vi "Process.vi"(8 "error in":errorcluster, 11 "Inst UI.Krohn-Hite-7008":refnum<class "Inst UI.Krohn-Hite-7008.lvclass">) -> (0 "error out":errorcluster, 3 "Inst UI.Krohn-Hite-7008 out":refnum<class "Inst UI.Krohn-Hite-7008.lvclass">)   [LabVIEW 2019, in "Inst.KH7008.lvlib" / "Inst UI.Krohn-Hite-7008.lvclass"]
doc: "---------------------------------------------------------------\nJKI State Machine Objects™\nhttp://jki.net/state-machine-objects/\nCopyright (C) 2005-2015, JKI <info@jki.net>\nALL RIGHTS RESERVEDJKI State Machine Objects (SMO) 1.0.0.5\nJKI - JKI\nCopyright (c) 2016, JKI"
uses:
  Inst UI.Krohn-Hite-7008.lvclass
  C:/Program Files/National Instruments/LabVIEW 2019/vi.lib/JKI/JKI SMO/SMO/SMO.lvclass
  C:/Program Files/National Instruments/LabVIEW 2019/user.lib/LevyLab/Instrument Framework/Instrument UI/Instrument UI.lvclass
  C:/Program Files/National Instruments/LabVIEW 2019/vi.lib/JKI/JKI SMO/SMO.UI/SMO.UI.lvclass
  KH7008/typedefs/allChannelProperties--Array.ctl
  KH7008/typedefs/channelProperties--Cluster.ctl
  KH7008/typedefs/channel--numeric.ctl
  KH7008/typedefs/gain--enum.ctl
  KH7008/typedefs/Input--Enum.ctl
  KH7008/typedefs/shunt--enum.ctl
  KH7008/typedefs/couple--Enum.ctl
  KH7008/typedefs/Filter--Enum.ctl
  Inst.Krohn-Hite-7008/Typedefs/setAllChannelsRequest--Cluster.ctl
  Inst.Krohn-Hite-7008/Inst.Krohn-Hite-7008.lvclass
  C:/Program Files/National Instruments/LabVIEW 2019/user.lib/LevyLab/Instrument Framework/Instrument/Instrument.lvclass
  <userlib>/LevyLab/Configuration/Configuration.lvclass
  <userlib>/LevyLab/RemoteControl/RemoteControl/Typedefs/Message--Cluster.ctl
  Inst.Krohn-Hite-7008/Typedefs/Inst.KH7008.device--Cluster.ctl
  <userlib>/LevyLab/Instrument Framework/Instrument UI/Instrument UI.lvclass/Instrument UI.ctl
  Inst UI.KH7008.UI--Cluster.ctl
  Inst.Krohn-Hite-7008/Typedefs/Inst.KH7008.getAll--Cluster.ctl
  Inst.Krohn-Hite-7008/Typedefs/getAllChannelsResponse--Cluster.ctl
  Inst.Krohn-Hite-7008/Inst.Krohn-Hite-7008.lvclass/Inst.Krohn-Hite-7008.ctl
  <vilib>/JKI/JKI SMO/SMO/SMO.lvclass/SMO.ctl
  <userlib>/LevyLab/Configuration/Configuration.lvclass/Configuration.ctl
  <userlib>/LevyLab/Instrument Framework/Instrument/Typedefs/Client Type--Enum.ctl
  <userlib>/LevyLab/Instrument Framework/Instrument/Instrument.lvclass/Instrument.ctl
  05e2a320-c8bb-41b2-9e77-26c6b753b84f.vi
  05e2a320-c8bb-41b2-9e77-26c6b753b84f.vi/d1df4cf9-d74a-44fa-a3ad-a094c8633207.vi
  05e2a320-c8bb-41b2-9e77-26c6b753b84f.vi/ff02851b-1958-46bb-bf4c-5be60d5017db.vi
  <vilib>/JKI/JKI SMO/SMO/Private/ReftoDVR--SMO.vi
  <vilib>/Utility/Data Type/Get Type Information.vi
  <vilib>/JDP Science/JSONtext/JSON text to Variant.vi
  <userlib>/LevyLab/Instrument Framework/Instrument/API/Instrument.sendMessageToProcess (variant).vi
  <vilib>/JDP Science/JSONtext/LVClass Serializer/JSONtext LVClass Serializer.lvclass
  <userlib>/LevyLab/Instrument Framework/Instrument/Instrument.lvclass
  <userlib>/LevyLab/Instrument Framework/Instrument UI/Instrument UI.lvclass
  <userlib>/LevyLab/RemoteControl/RemoteControl/RemoteControl.lvclass
  KH7008/KH7008.lvlib
  <vilib>/JKI/JKI SMO/SMO.UI/SMO.UI.lvclass
  <vilib>/JKI/JKI SMO/SMO/SMO.lvclass
  C:/Program Files/National Instruments/LabVIEW 2019/user.lib/LevyLab/Instrument Framework/Instrument Types/Amplifier/Instrument.Amplifier.lvclass
panel:
  out "String":string
  out "Slide":i32(slide) scale=0.0..60000.0
  in  "Cancel":bool
  in  "allChannelProperties":T1 {"channel" min=1 max=8 step=1}
  out "device":string
  out "Numeric":u32
  in  "Update":bool
  in  "STOP":bool
  # "SMO UI Template"
  # "For instructions on how to use the JKI State Machine Objects, examples and video tutorials, visit:\nhttp://jki.net/state-machine-objects/\n\nJKI State Machine Objects™\nhttp://jki.net/state-machine-objects/\nCopyright (C) 2005-2015, JKI <info@jki.net>\nALL RIGHTS RESERVED"
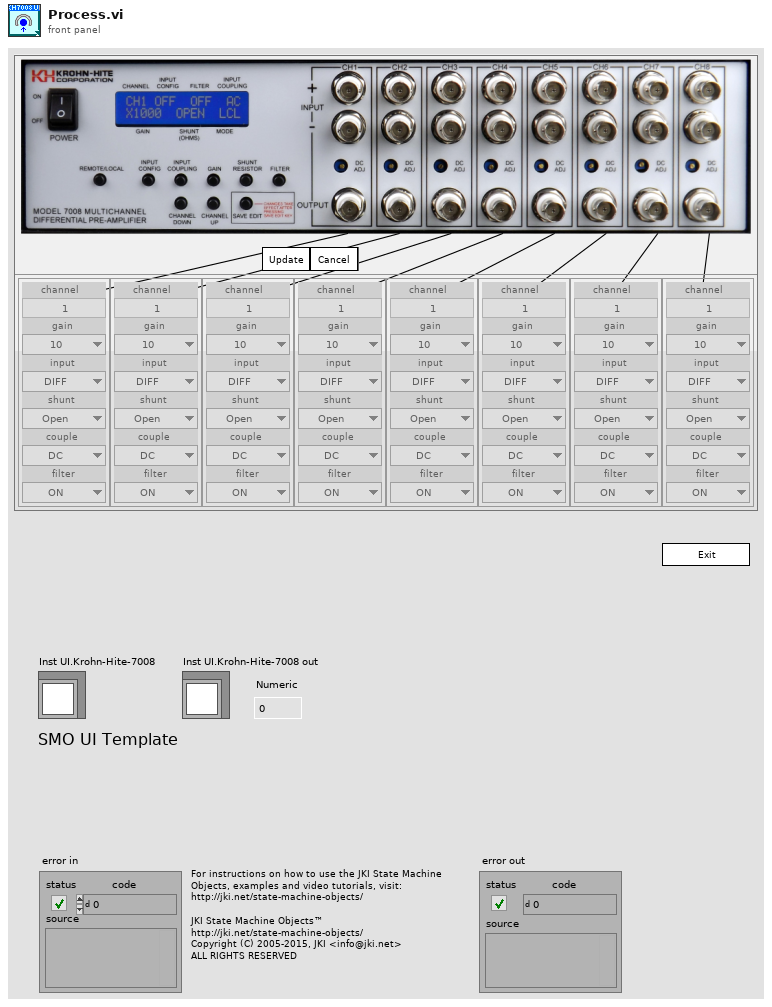
[diagram p1: front panel]
types:
  T1 = typedef "KH7008.lvlib/allChannelProperties--Array.ctl" = T2[]
  T2 = typedef "KH7008.lvlib/channelProperties--Cluster.ctl" = cluster{"channel":T3, "gain":T4, "input":T5, "shunt":T6, "couple":T7, "filter":T8}
  T3 = typedef "KH7008.lvlib/channel--numeric.ctl" = u16
  T4 = typedef "KH7008.lvlib/gain--enum.ctl" = enum16{"1", "10", "100", "1000"}
  T5 = typedef "KH7008.lvlib/input--enum.ctl" = enum16{"OFF", "SE+", "SE-", "DIFF"}
  T6 = typedef "KH7008.lvlib/shunt--enum.ctl" = enum16{"Open", "50", "500", "5k", "50k", "10M"}
  T7 = typedef "KH7008.lvlib/couple--enum.ctl" = enum16{"AC", "DC"}
  T8 = typedef "KH7008.lvlib/filter--enum.ctl" = enum16{"OFF", "ON"}
  T9 = typedef "Inst.KH7008.lvlib/Inst.Krohn-Hite-7008.lvclass/setAllChannelsRequest--Cluster.ctl" = cluster{"allChannelProperties":T1}
  T10 = enum32{"invalid app kind", "Development System", "Run Time System", "Student Edition", "Embedded LabVIEW", "Evaluation", "Custom"}
  T11 = typedef "Inst.KH7008.lvlib/Inst.Krohn-Hite-7008.lvclass/getAllChannelsResponse--Cluster.ctl" = cluster{"allChannelProperties":T1}
  T12 = enum32{"Invalid", "Standard", "Closed", "Hidden", "Minimized", "Maximized"}
  T13 = typedef "Instrument.lvlib/Instrument.lvclass/Client Type--Enum.ctl" = enum16{"Remote", "Local"}
  T14 = typedef "RemoteControl.lvlib/RemoteControl.lvclass/Message--Cluster.ctl" = cluster{"Command":string, "Data":variant, "ID":string}
  T15 = typedef "Inst.KH7008.lvlib/Inst.Krohn-Hite-7008.lvclass/Inst.KH7008.device--Cluster.ctl" = cluster{"model":string, "device_id":string, "index":i32}
  T16 = cluster{"Core":cluster{"Current VI Reference":refnum<vi>, "Close Panel on Exit?":bool, "Last Error":cluster{"error":errorcluster, "previous state":string, "remaining states":string}, "Shutdown?":bool}, "Instrument UI":refnum<class "Inst UI.Krohn-Hite-7008.lvclass">, "Instrument":refnum<class "Inst.Krohn-Hite-7008.lvclass">, "Configuration":refnum<class "Configuration.lvclass">, "Message":T14, "allChannelProperties":T1, "Device":T15, "Edit State":bool, "Timer Reset":bool}
  T17 = typedef "RemoteControl.lvclass/Message--Cluster.ctl" = cluster{"Command":string, "Data":variant, "ID":string}
  T18 = typedef "Inst.KH7008.lvlib/Inst.Krohn-Hite-7008.lvclass/Inst.KH7008.getAll--Cluster.ctl" = cluster{"allChannelProperties":T1}
  T19 = typedef "Inst.KH7008.lvlib/Inst UI.Krohn-Hite-7008.lvclass/Inst UI.KH7008.UI--Cluster.ctl" = cluster{"setAllChannelsRequest":T9}
  T20 = cluster{"Current VI Reference":refnum<vi>, "Close Panel on Exit?":bool, "Last Error":cluster{"error":errorcluster, "previous state":string, "remaining states":string}, "Shutdown?":bool}
  T21 = typedef "SMO.lvclass/Protected Events.ctl" = cluster{"StopProcesses":refnum<user-event>, "AbortProcesses":refnum<user-event>, "Config Changed":refnum<user-event>, "Dependency":refnum<user-event>}
  T22 = typedef "Instrument.lvlib/Instrument.lvclass/PublicEvents--Cluster.ctl" = cluster{"MessageFromProcess":refnum<user-event>}
  T23 = typedef "Inst.KH7008.lvlib/Inst.Krohn-Hite-7008.lvclass/PublicEvents--Cluster.ctl" = cluster{"MessageFromProcess":refnum<user-event>}
  T24 = typedef "Instrument.lvlib/Instrument.lvclass/Instrument.IDN--cluster.ctl" = cluster{"vendor":string, "model":string, "serial":string, "firmware":string}
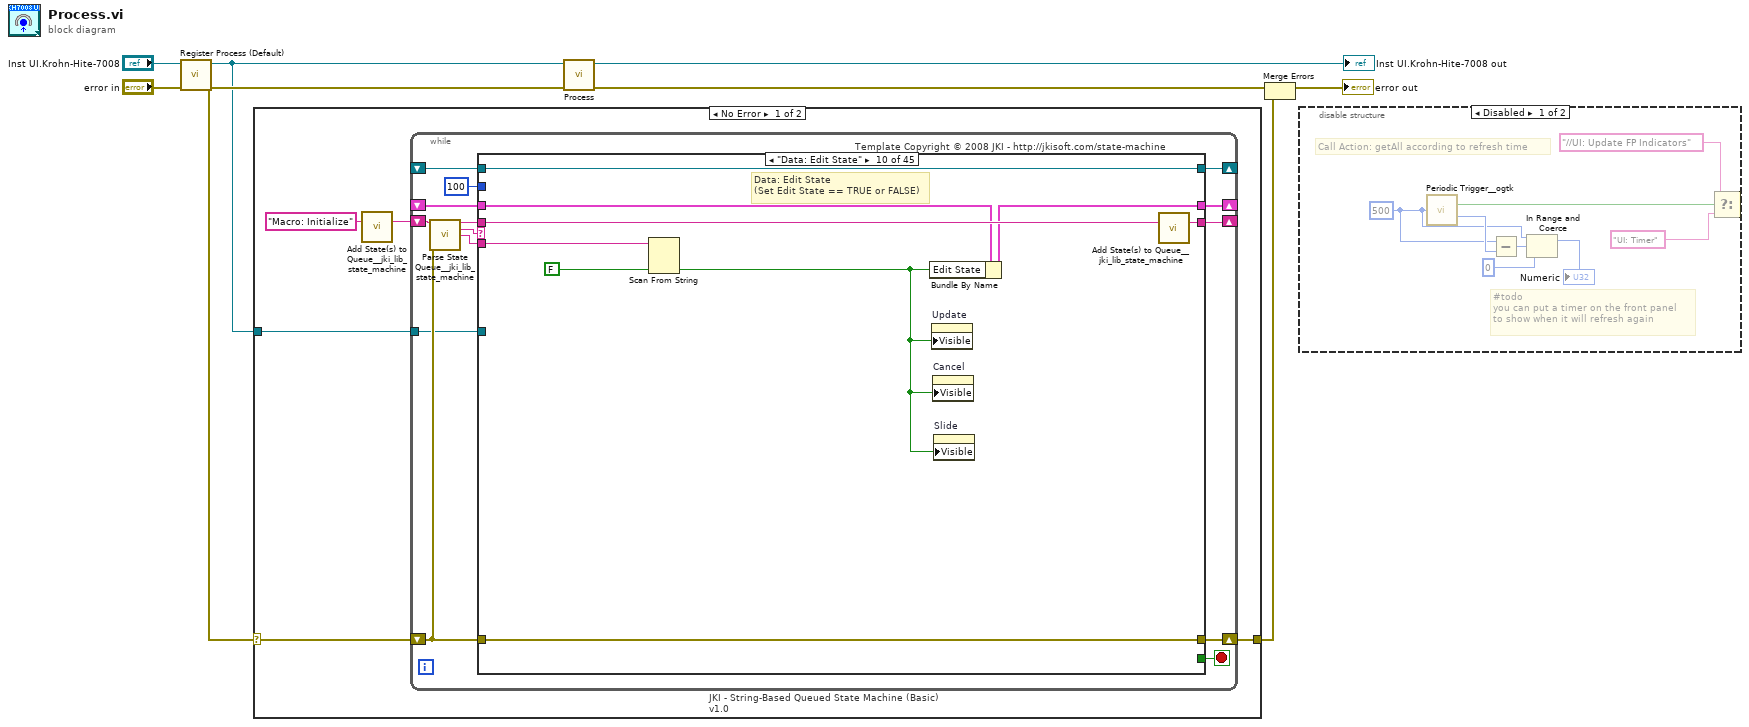
[diagram p0: block diagram]
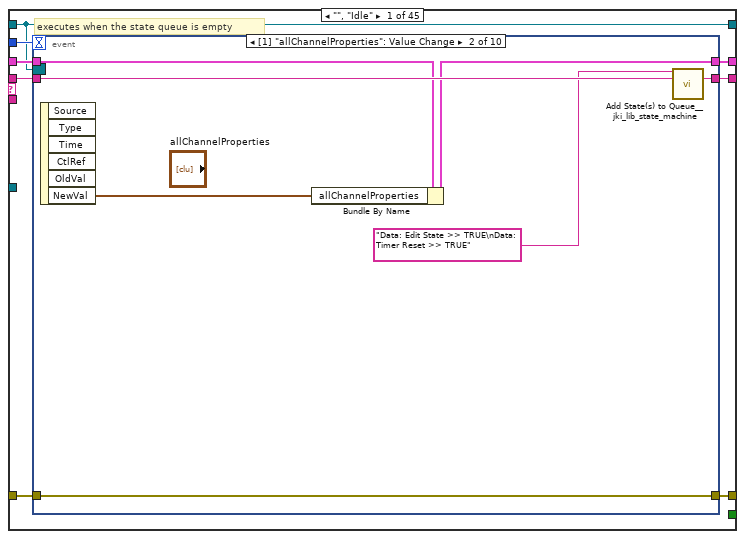
[diagram p3: hidden frame]
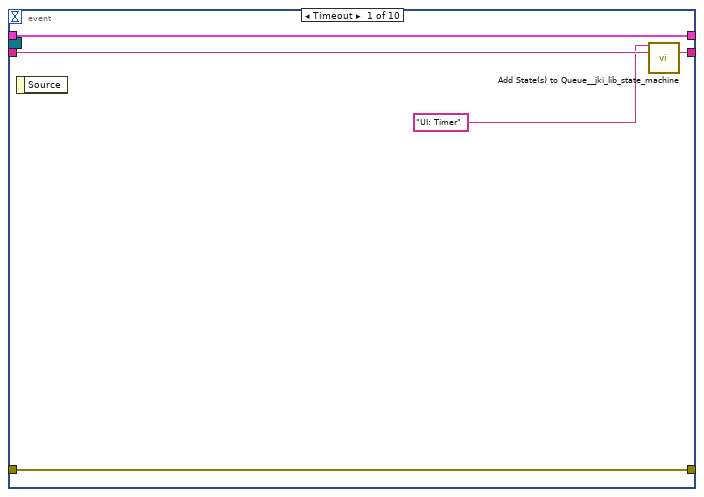
[diagram p4: hidden frame]
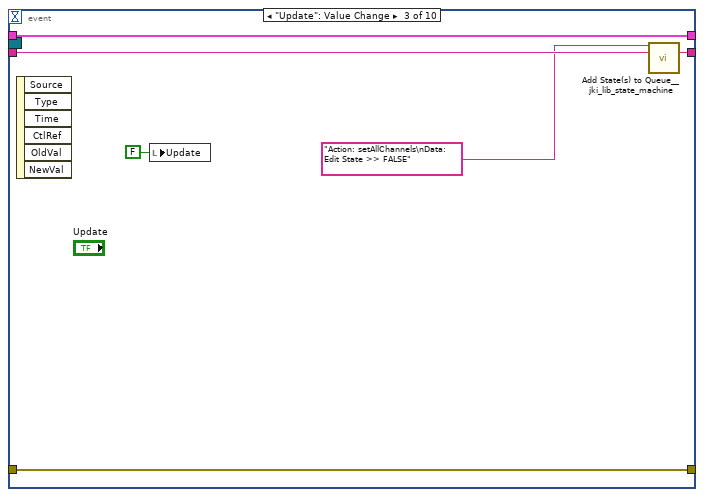
[diagram p5: hidden frame]
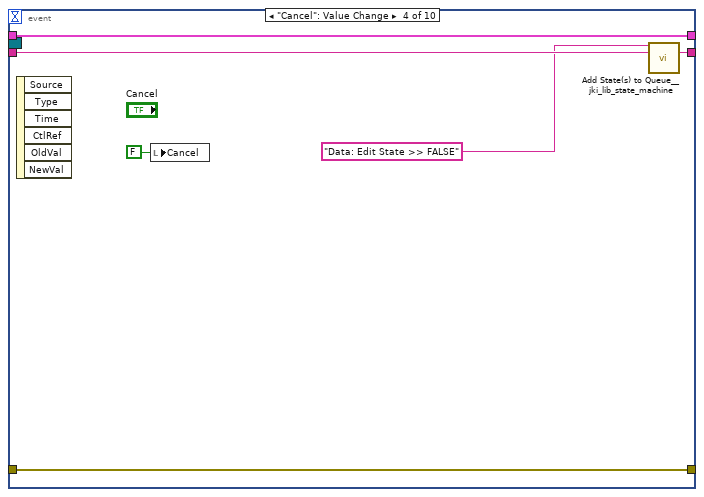
[diagram p6: hidden frame]
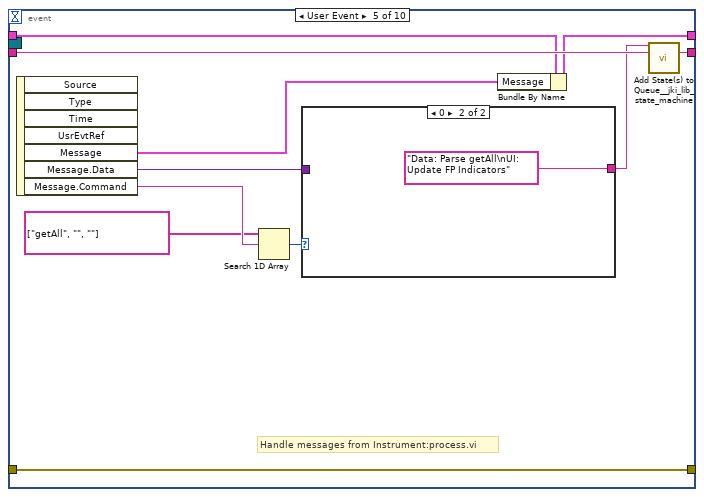
[diagram p7: hidden frame]
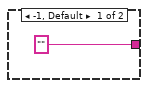
[diagram p8: hidden frame]
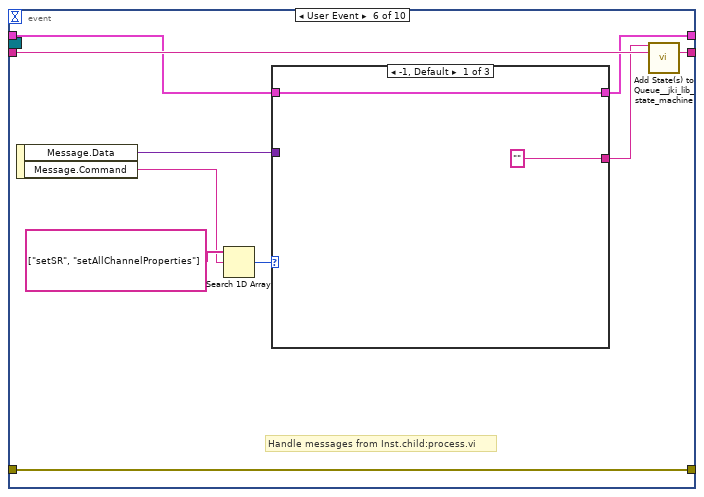
[diagram p9: hidden frame]
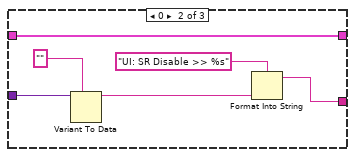
[diagram p10: hidden frame]
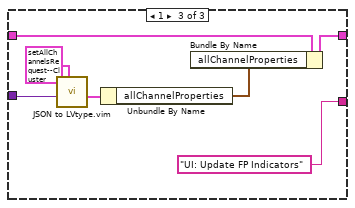
[diagram p11: hidden frame]
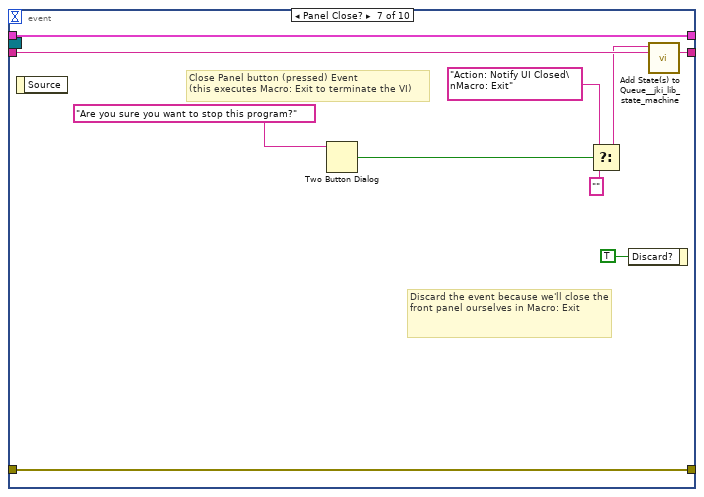
[diagram p12: hidden frame]
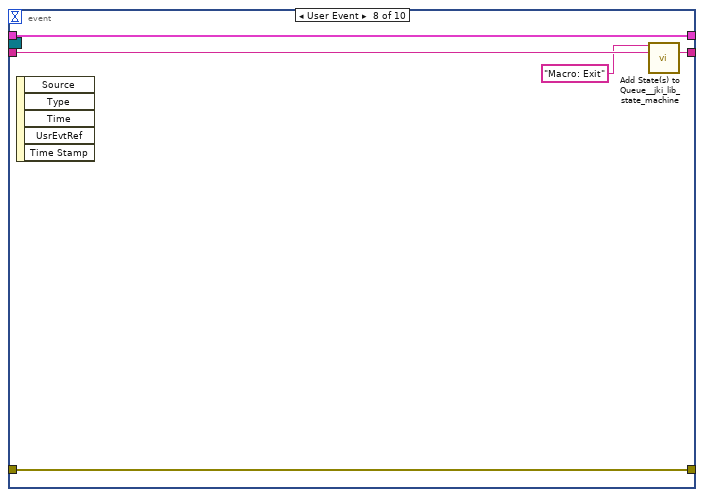
[diagram p13: hidden frame]
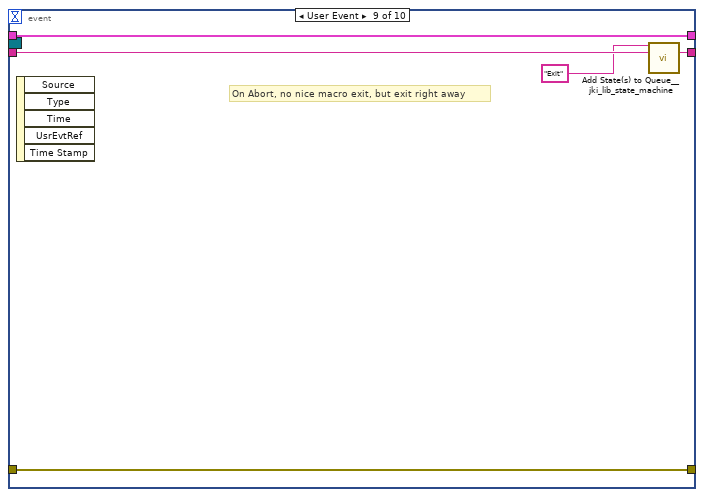
[diagram p14: hidden frame]
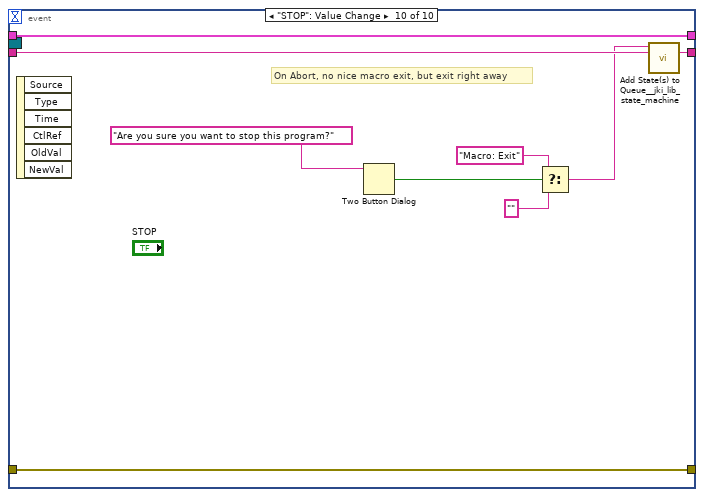
[diagram p15: hidden frame]
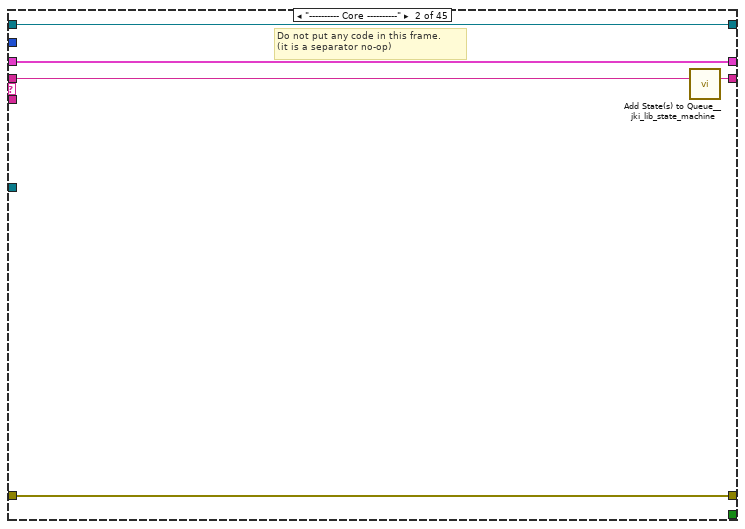
[diagram p16: hidden frame]
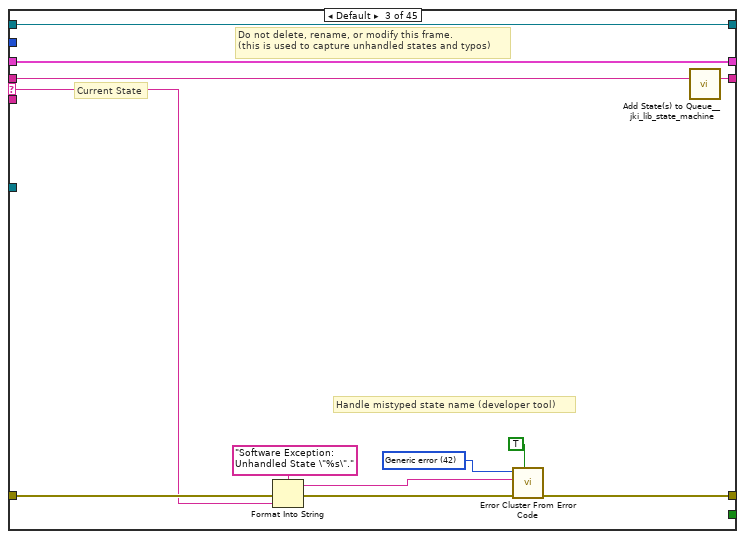
[diagram p17: hidden frame]
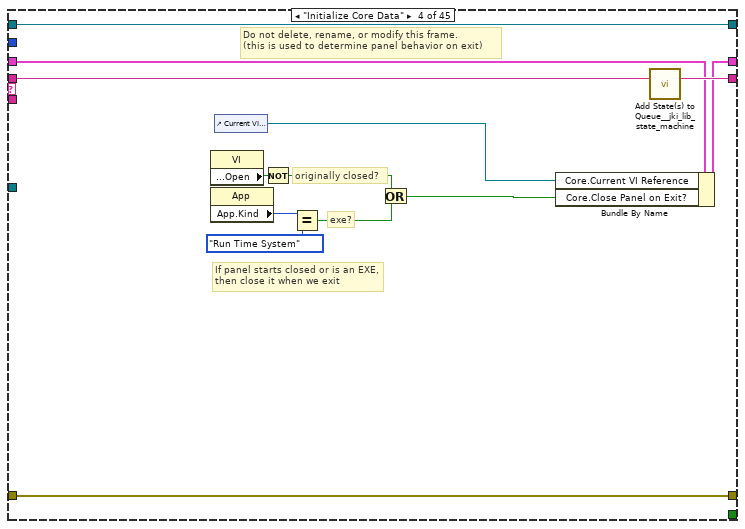
[diagram p18: hidden frame]
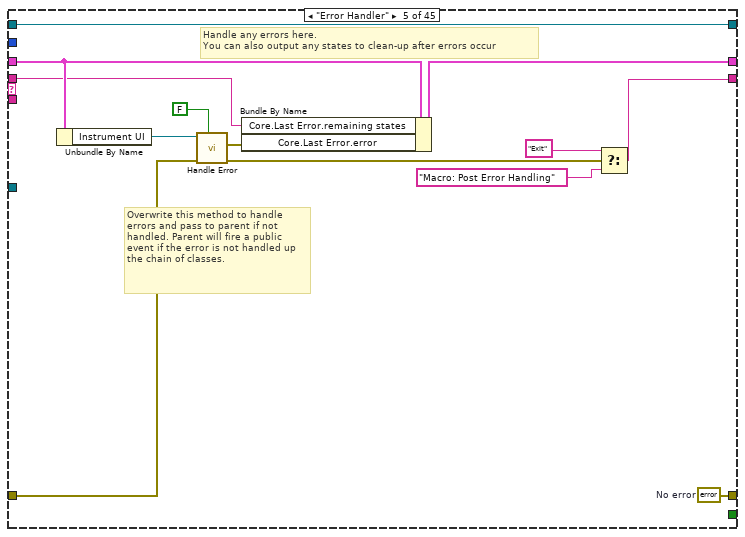
[diagram p19: hidden frame]
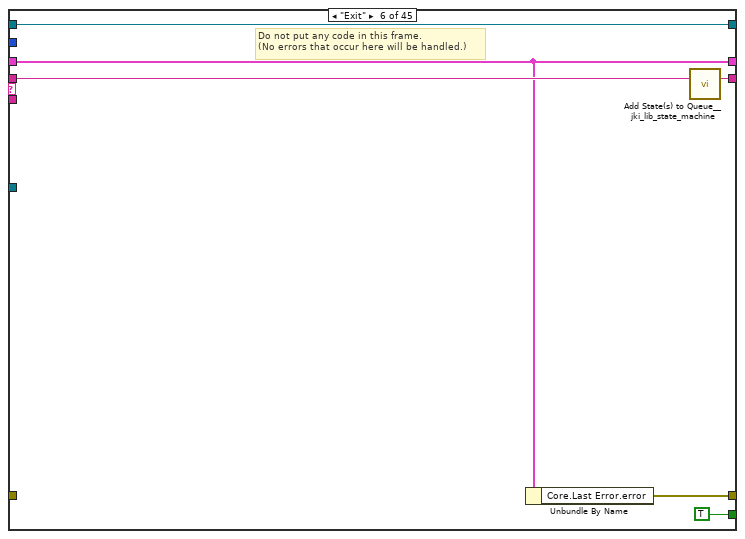
[diagram p20: hidden frame]
diagram:
  n1 = call <vilib>:"Register Process (Default).vi"("error in (no error)"="error in", "SMO"="Inst UI.Krohn-Hite-7008") -> ("error out"=w5:errorcluster, "SelfRef"=w4:refnum<class "Inst UI.Krohn-Hite-7008.lvclass">)  [unwired: 8 in]
  n2 = case shown="No Error" w5 {
    selector: w5 -> [w10 w608]
    tunnel: w4 -> [w11 _]
    tunnel: [w9 w608] -> w1
    frame No Error {
      n3 = call <vilib>:"Add State(s) to Queue__jki_lib_state_machine.vi"("State(s) in (\"\")"="Macro: Initialize") -> ("States Out"=w13:string)  [unwired: 14 in]
      n4 = while "JKI - String-Based Queued State Machine (Basic) v1.0" {
        shift-right: [w21] -> _
        shift-left: _ -> [w20]
        shift-right: [w24] -> w9
        shift-left: w10 -> [w18]
        shift-right: [w23] -> _
        shift-left: w13 -> [w25]
        tunnel: w11 -> [w17]
        shift-right: [w16] -> _
        shift-left: _ -> [w15]
        stop <- w22 stop-if-true
        # "Template Copyright © 2008 JKI - http://jkisoft.com/state-machine"
        n5 = call <vilib>:"Parse State Queue__jki_lib_state_machine.vi"("State Queue"=w25, "Error In (no error)"=w18) -> ("Remaining States"=w27:string, "Current State"=w14:string, "Arguments"=w26:string)  [unwired: 11 in]
        n6 = case shown="\"Data: Edit State\"" w14 {
          selector: w14 -> [_ _ w133 _ _ _ _ _ _ _ _ _ _ _ _ _ _ _ _ _ _ _ _ _ _ _ _ _ _ _ _ _ _ _ _ _ _ _ _ _ _ _ _ _ _]
          tunnel: w27 -> [w35 w131 w137 w156 w160 w175 w180 w199 w204 w213 w222 w233 w248 w253 w261 w276 w301 w313 w325 w341 w373 w382 w394 w404 w410 w425 w430 w441 w448 w453 w469 w475 w480 w495 w503 w515 w522 w529 w542 w555 w565 w576 w587 w597 w607]
          tunnel: w26 -> [_ _ _ _ _ _ _ _ _ w209 w218 _ _ _ _ _ _ w306 w319 w335 _ _ _ _ _ _ _ _ _ _ _ _ _ _ _ _ _ _ _ _ _ w566 _ _ _]
          tunnel: w20 -> [w33 w128 w135 w147 w163 w171 w177 _ w200 w206 w214 w224 w242 w250 w259 w273 w289 w307 w323 w337 w370 w378 w384 w401 w407 w412 w427 w438 w443 w450 w467 w473 w477 w488 w500 w506 w517 w523 w536 w552 w557 w571 w582 w592 w602]
          tunnel: [w32 w129 w139 w153 w165 w170 w178 w192 w202 w211 w220 w228 w244 w251 w256 w265 w299 w309 w320 w338 w371 w380 w392 w402 w408 w423 w428 w432 w444 w451 w464 w470 w478 w481 w498 w507 w519 w524 w539 w548 w562 w573 w579 w588 w598] -> w24
          tunnel: w18 -> [w31 w129 w138 w153 w159 _ w178 w181 w202 w211 w220 w227 w245 w251 w257 w264 w299 w308 w321 w339 w371 w380 w392 w402 w408 w423 w428 w433 w445 w451 w454 w471 w478 w490 w496 w508 w519 w525 w531 w547 w558 w573 w580 w589 w599]
          tunnel: [w34 w130 w136 w155 w157 w174 w179 w198 w203 w212 w221 w232 w247 w252 w260 w275 w300 w312 w324 w340 w372 w381 w393 w403 w409 w424 w429 w440 w447 w452 w468 w474 w479 w494 w502 w514 w521 w528 w541 w554 w564 w575 w586 w596 w606] -> w23
          tunnel: [_ _ _ _ _ TRUE _ _ _ _ _ _ _ _ _ _ _ _ _ _ _ _ _ _ _ _ _ _ _ _ _ _ _ _ _ _ _ _ _ _ _ _ _ _ _] -> w22
          tunnel: [w30 w128 w135 w154 w162 w171 w177 w197 w200 w207 w215 w229 w242 w250 w259 w273 w289 w307 w323 w337 w370 w378 w385 w401 w407 w412 w427 w438 w443 w450 w467 w473 w477 w492 w500 w504 w516 w523 w537 w551 w559 w570 w583 w593 w603] -> w21
          tunnel: 100 ("Timeout") -> [w29 _ _ _ _ _ _ _ _ _ _ _ _ _ _ _ _ _ _ _ _ _ _ _ _ _ _ _ _ _ _ _ _ _ _ _ _ _ _ _ _ _ _ _ _]
          tunnel: w17 -> [_ _ _ _ _ _ _ w184 _ _ _ _ _ _ _ _ _ _ _ _ _ _ _ _ _ _ _ _ _ _ _ _ _ _ _ _ _ _ _ _ _ _ _ _ _]
          tunnel: [w28 w127 w132 w144 w169 w172 w176 w196 w201 w210 w219 w231 w243 w249 w258 w274 w298 w311 w322 w334 w369 w379 w391 w400 w406 w417 w426 w439 w446 w449 w466 w472 w476 w493 w501 w513 w520 w527 w540 w553 w563 w574 w585 w595 w605] -> w16
          tunnel: w15 -> [w28 w127 w132 w144 w169 w172 w176 w196 w201 w210 w219 w231 w243 w249 w258 w274 w298 w311 w322 w334 w369 w379 w391 w400 w406 w417 w426 w439 w446 w449 _ w472 w476 w493 w501 w513 w520 w527 w540 w553 w563 w574 w585 w595 w605]
          frame "", "Idle" {
            # "executes when the state queue is empty"
            n7 = event shown="[1] \"allChannelProperties\": Value Change" {
              selector: w28 -> [_ _ _ _ _ _ _ _ _ _]
              dyn-events: _ -> [_ _ _ _ _ _ _ _ _ _]
              timeout: w29 -> [_ _ _ _ _ _ _ _ _ _]
              tunnel: w35 -> [w40 w47 w53 w59 w70 w82 w107 w112 w117 w126]
              tunnel: [w39 w46 w52 w58 w69 w81 w106 w111 w116 w125] -> w34
              tunnel: w33 -> [w37 w41 w50 w56 w66 w73 w104 w109 w114 w123]
              tunnel: [w38 w45 w51 w57 w68 w80 w103 w110 w115 w124] -> w32
              tunnel: w31 -> [w38 w45 w51 w57 w68 w80 w103 w110 w115 w124]
              tunnel: [w37 w42 w50 w56 w62 w74 w104 w109 w114 w123] -> w30
              event Timeout {
                n8 = event-data() -> ()  [unwired: 1 in, 1 out]
                n9 = call <vilib>:"Add State(s) to Queue__jki_lib_state_machine.vi"("State(s) in Front (\"\")"="UI: Timer" ("State(s) in Front (\"\")"), "State(s) in (\"\")"=w40) -> ("States Out"=w39:string)  [unwired: 13 in]
              }
              event Value Change {
                n10 = event-data() -> ("NewVal"=w43:T1)  [unwired: 1 in, 5 out]
                n11 = Bundle By Name(cluster=w41, "allChannelProperties"=w43) -> (w42:T16)
                n12 = call <vilib>:"Add State(s) to Queue__jki_lib_state_machine.vi"("State(s) in Front (\"\")"="Data: Edit State >> TRUE\nData: Timer Reset >> TRUE" ("State(s) in Front (\"\")"), "State(s) in (\"\")"=w47) -> ("States Out"=w46:string)  [unwired: 13 in]
              }
              event "Update": Value Change {
                n13 = event-data() -> ()  [unwired: 1 in, 6 out]
                n14 = local write "Update"(FALSE ("Update")) -> ()
                n15 = call <vilib>:"Add State(s) to Queue__jki_lib_state_machine.vi"("State(s) in Front (\"\")"="Action: setAllChannels\nData: Edit State >> FALSE" ("State(s) in Front (\"\")"), "State(s) in (\"\")"=w53) -> ("States Out"=w52:string)  [unwired: 13 in]
              }
              event "Cancel": Value Change {
                n16 = event-data() -> ()  [unwired: 1 in, 6 out]
                n17 = local write "Cancel"(FALSE ("Cancel")) -> ()
                n18 = call <vilib>:"Add State(s) to Queue__jki_lib_state_machine.vi"("State(s) in Front (\"\")"="Data: Edit State >> FALSE" ("State(s) in Front (\"\")"), "State(s) in (\"\")"=w59) -> ("States Out"=w58:string)  [unwired: 13 in]
              }
              event User Event {
                # "Handle messages from Instrument:process.vi"
                n19 = event-data() -> ("Message"=w61:T17, "Message.Data"=w64:variant, "Message.Command"=w67:string)  [unwired: 1 in, 4 out]
                n20 = Search 1D Array(1D array=string[] ["getAll", "", ""], element=w67) -> (index of element=w65:i32)  [unwired: 1 in]
                n21 = case shown="0" w65 {
                  tunnel: ["" ("State(s) in Front (\"\")") "Data: Parse getAll\nUI: Update FP Indicators" ("State(s) in Front (\"\")")] -> w60
                  tunnel: w64 -> [_ _]
                  frame -1, Default {
                  }
                  frame 0 {
                  }
                }
                n22 = Bundle By Name(cluster=w66, "Message"=w61) -> (w62:T16)
                n23 = call <vilib>:"Add State(s) to Queue__jki_lib_state_machine.vi"("State(s) in Front (\"\")"=w60, "State(s) in (\"\")"=w70) -> ("States Out"=w69:string)  [unwired: 13 in]
              }
              event User Event {
                # "Handle messages from Inst.child:process.vi"
                n24 = event-data() -> ("Message.Data"=w75:variant, "Message.Command"=w77:string)  [unwired: 1 in]
                n25 = Search 1D Array(1D array=string[] ["setSR", "setAllChannelProperties"], element=w77) -> (index of element=w76:i32)  [unwired: 1 in]
                n26 = case shown="-1, Default" w76 {
                  tunnel: ["" ("State(s) in Front (\"\")") w88 "UI: Update FP Indicators" ("State(s) in Front (\"\")")] -> w79
                  tunnel: w75 -> [_ w85 w92]
                  tunnel: w73 -> [w83 w86 w96]
                  tunnel: [w83 w86 w95] -> w74
                  frame -1, Default {
                  }
                  frame 0 {
                    n27 = Variant To Data(type="", Variant=w85) -> (data=w89:string)  [unwired: 1 in, 1 out]
                    n28 = Format Into String(format string="UI: SR Disable >> %s" ("State(s) in Front (\"\")"), w89) -> (resulting string=w88:string)  [unwired: 2 in, 1 out]
                  }
                  frame 1 {
                    n29 = call "JSON to LVtype.vim"("type"=T9 {"allChannelProperties"=[{"channel"=1, "gain"=enum."10", "input"=enum."OFF", "shunt"=enum."10M", "couple"=enum."AC", "filter"=enum."OFF"}, {"channel"=2, "gain"=enum."10", "input"=enum."OFF", "shunt"=enum."10M", "couple"=enum."AC", "filter"=enum."OFF"}, {"channel"=3, "gain"=enum."10", "input"=enum."OFF", "shunt"=enum."10M", "couple"=enum."AC", "filter"=enum."OFF"}, {"channel"=4, "gain"=enum."10", "input"=enum."OFF", "shunt"=enum."10M", "couple"=enum."AC", "filter"=enum."OFF"}, {"channel"=5, "gain"=enum."10", "input"=enum."OFF", "shunt"=enum."10M", "couple"=enum."AC", "filter"=enum."OFF"}, {"channel"=6, "gain"=enum."10", "input"=enum."OFF", "shunt"=enum."10M", "couple"=enum."AC", "filter"=enum."OFF"}, {"channel"=7, "gain"=enum."10", "input"=enum."OFF", "shunt"=enum."10M", "couple"=enum."AC", "filter"=enum."OFF"}, {"channel"=7, "gain"=enum."10", "input"=enum."OFF", "shunt"=enum."10M", "couple"=enum."AC", "filter"=enum."OFF"}]} ("setAllChannelsRequest"), "JSON Data in"=w92) -> ("Data out"=w94:T9)  [unwired: 8 in, 1 out]
                    n30 = Unbundle By Name(w94) -> ("allChannelProperties"=w93:T1)
                    n31 = Bundle By Name(cluster=w96, "allChannelProperties"=w93) -> (w95:T16)
                  }
                }
                n32 = call <vilib>:"Add State(s) to Queue__jki_lib_state_machine.vi"("State(s) in Front (\"\")"=w79, "State(s) in (\"\")"=w82) -> ("States Out"=w81:string)  [unwired: 13 in]
              }
              event Panel Close? {
                # "Discard the event because we'll close the front panel ourselves in Macro: Exit"
                # "Close Panel button (pressed) Event\n(this executes Macro: Exit to terminate the VI)"
                n33 = event-data() -> ()  [unwired: 1 in, 1 out]
                n34 = Two Button Dialog(message="Are you sure you want to stop this program?") -> (T button?=w102:bool)  [unwired: 2 in]
                n35 = Select(t="Action: Notify UI Closed\nMacro: Exit", s=w102, f="") -> (s? t:f=w98:string)
                n36 = event-data("Discard?"=TRUE) -> ()  [unwired: 1 in, 1 out]
                n37 = call <vilib>:"Add State(s) to Queue__jki_lib_state_machine.vi"("State(s) in Front (\"\")"=w98, "State(s) in (\"\")"=w107) -> ("States Out"=w106:string)  [unwired: 13 in]
              }
              event User Event {
                n38 = event-data() -> ()  [unwired: 1 in, 5 out]
                n39 = call <vilib>:"Add State(s) to Queue__jki_lib_state_machine.vi"("State(s) in Front (\"\")"="Macro: Exit", "State(s) in (\"\")"=w112) -> ("States Out"=w111:string)  [unwired: 13 in]
              }
              event User Event {
                # "On Abort, no nice macro exit, but exit right away"
                n40 = event-data() -> ()  [unwired: 1 in, 5 out]
                n41 = call <vilib>:"Add State(s) to Queue__jki_lib_state_machine.vi"("State(s) in Front (\"\")"="Exit", "State(s) in (\"\")"=w117) -> ("States Out"=w116:string)  [unwired: 13 in]
              }
              event "STOP": Value Change {
                # "On Abort, no nice macro exit, but exit right away"
                n42 = event-data() -> ()  [unwired: 1 in, 6 out]
                n43 = Two Button Dialog(message="Are you sure you want to stop this program?") -> (T button?=w122:bool)  [unwired: 2 in]
                n44 = Select(t="Macro: Exit", s=w122, f="") -> (s? t:f=w118:string)
                n45 = call <vilib>:"Add State(s) to Queue__jki_lib_state_machine.vi"("State(s) in Front (\"\")"=w118, "State(s) in (\"\")"=w126) -> ("States Out"=w125:string)  [unwired: 13 in]
              }
            }
          }
          frame "---------- Core ----------" {
            # "Do not put any code in this frame.\n(it is a separator no-op)"
            n46 = call <vilib>:"Add State(s) to Queue__jki_lib_state_machine.vi"("State(s) in (\"\")"=w131) -> ("States Out"=w130:string)  [unwired: 14 in]
          }
          frame Default {
            w142 = 42 items=["No error", "Argument error", "Memory is full", "Out of zone", "End of file", "File already open", "Generic file I/O error", "File not found", "File permission error", "Disk is full", "Duplicate path", "Too many files open", "System feature not enabled", "Resource file not found", "Cannot add resource", "Resource not found", "Image not found", "Image memory error", "Pen does not exist", "Config type invalid", "Config token not found", "Config parse error", "Config memory error", "Bad external code format", "Bad external code offset", "External code not present", "Null window", "Destroy window error", "Null menu", "Print aborted", "Bad print record", "Print driver error", "Windows error during printing", "Memory error during printing", "Print dialog error", "Generic print error", "Invalid device refnum", "Device not found", "Device parameter error", "Device unit error", "Cannot open device", "Device call aborted", "Generic error", "Cancelled by user", "Object ID too low", "Object ID too high", "Object not in heap", "Unknown heap", "Unknown object (invalid DefProc)", "Unknown object (DefProc not in table)", "Message out of range", "Invalid (null) method", "Unknown message", "Manager call not supported", "Bad address", "Network operation in progress", "Network operation timed out", "Connection is busy", "Network attribute not supported", "Network error", "Address in use", "System out of memory", "Connection aborted", "Connection refused", "Not connected", "Already connected", "Connection closed", "Initialization error (interapplication manager)", "Bad occurrence", "Wait on unbound occurrence handler", "Occurrence queue overflow", "Datalog type conflict", "Unused", "Unrecognized type (interapplication manager)", "Memory corrupt", "Failed to make temporary DLL", "Old CIN version", "Drag socket not found", "Failed to load drop-object", "Failed to register OLE object", "Failed to release OLE object", "Format specifier type mismatch", "Unknown format specifier", "Too few format specifiers", "Too many format specifiers", "Scan failed", "Newer CIN version", "Error converting to variant", "Runtime menu error", "Password tampered", "Variant attribute not found", "Incompatible variant data type", "Event data is not available", "Event Store is not present", "Occurrence is not found", "Event Queue is not created", "Event info is not available", "Refnum passed is NULL", "Error retrieving Class GUID", "Error retrieving CoClass GUID", "Error retrieving TypeLib GUID.", "Bad built application magic bytes.", "Specific driver is different from the specific driver associated with the Logical Name.", "There is no session opened to the class driver.", "Max Error", "MAX - Error with config objects", "MAX - Error loading configuration", "MAX - Group not supported"]
            # "Current State"
            # "Do not delete, rename, or modify this frame.\n(this is used to capture unhandled states and typos)"
            # "Handle mistyped state name (developer tool)"
            n47 = Format Into String(format string="Software Exception: Unhandled State \"%s\"." ("message"), error in=w138, w133) -> (resulting string=w141:string, error out=w140:errorcluster)  [unwired: 1 in]
            n48 = call <vilib>:"Error Cluster From Error Code.vi"("show call chain? (False)"=TRUE, "error in (no error)"=w140, "error message (\"\")"=w141, "error code (0)"=w142) -> ("error out"=w139:errorcluster)  [unwired: 5 in]
            n49 = call <vilib>:"Add State(s) to Queue__jki_lib_state_machine.vi"("State(s) in (\"\")"=w137) -> ("States Out"=w136:string)  [unwired: 14 in]
          }
          frame "Initialize Core Data" {
            # "Do not delete, rename, or modify this frame.\n(this is used to determine panel behavior on exit)"
            # "originally closed?"
            # "exe?"
            # "If panel starts closed or is an EXE, then close it when we exit"
            n50 = property class="VI"() -> ("Front Panel.Open"=w152:bool)  [unwired: 2 in, 2 out]
            n51 = property class="App"() -> ("App.Kind"=w151:T10)  [unwired: 2 in, 2 out]
            n52 = control-ref of="Current VI Reference"() -> (w145:refnum<vi>)
            n53 = Not(x=w152) -> (.not. x?=w149:bool)
            n54 = Equal?(x=w151, y=T10."Run Time System" ("Application:Kind")) -> (x = y?=w148:bool)
            n55 = Or(x=w149, y=w148) -> (x .or. y?=w146:bool)
            n56 = Bundle By Name(cluster=w147, "Core.Current VI Reference"=w145, "Core.Close Panel on Exit?"=w146) -> (w154:T16)
            n57 = call <vilib>:"Add State(s) to Queue__jki_lib_state_machine.vi"("State(s) in (\"\")"=w156) -> ("States Out"=w155:string)  [unwired: 14 in]
          }
          frame "Error Handler" {
            w165 = errorcluster {"status"=FALSE, "code"=0, "source"=""}  # No error
            # "Overwrite this method to handle errors and pass to parent if not handled. Parent will fire a public event if the error is not handled up the chain of classes."
            # "Handle any errors here.\nYou can also output any states to clean-up after errors occur"
            n58 = Unbundle By Name(w163) -> ("Instrument UI"=w168:refnum<class "Inst UI.Krohn-Hite-7008.lvclass">)
            n59 = call-dynamic "Handle Error.vi"("Stop on Unhandled Error (T)"=FALSE, "error in"=w159, "SMO"=w168) -> ("handling error"=w166:errorcluster, "Unhandled error"=w164:errorcluster)  [unwired: 6 in, 1 out]
            n60 = Bundle By Name(cluster=w163, "Core.Last Error.remaining states"=w160, "Core.Last Error.error"=w164) -> (w162:T16)
            n61 = Select(t="Exit", s=w166, f="Macro: Post Error Handling") -> (s? t:f=w157:string)
          }
          frame "Exit" {
            # "Do not put any code in this frame.\n(No errors that occur here will be handled.)"
            n62 = Unbundle By Name(w171) -> ("Core.Last Error.error"=w170:errorcluster)
            n63 = call <vilib>:"Add State(s) to Queue__jki_lib_state_machine.vi"("State(s) in (\"\")"=w175) -> ("States Out"=w174:string)  [unwired: 14 in]
          }
          frame "---------- Data ----------" {
            # "Do not put any code in this frame.\n(It is a separator no-op. You can make a copy of this frame to create a new Data frame)"
            n64 = call <vilib>:"Add State(s) to Queue__jki_lib_state_machine.vi"("State(s) in (\"\")"=w180) -> ("States Out"=w179:string)  [unwired: 14 in]
          }
          frame "Data: Initialize" {
            w186 = T15 {"model"="", "device_id"="", "index"=0}  # Device
            w187 = FALSE  # Timer Reset
            (unwired) T18 {"allChannelProperties"=[]}  # getAll
            w188 = FALSE  # Edit State
            w189 = T1 []  # allChannelProperties
            w190 = T14 {"Command"="", "Data"=variant, "ID"=""}  # Message
            w191 = refnum<class "Configuration.lvclass"> refnum  # Configuration
            (unwired) T19 {"setAllChannelsRequest"={"allChannelProperties"=[]}}  # UI Cluster
            w194 = refnum<class "Inst.Krohn-Hite-7008.lvclass"> refnum  # Instrument
            w195 = T20 {"Current VI Reference"=refnum, "Close Panel on Exit?"=FALSE, "Last Error"={"error"={"status"=FALSE, "code"=0, "source"=""}, "previous state"="", "remaining states"=""}, "Shutdown?"=FALSE}  # Core
            # "Cluster of UI\ninformation you\nwant to save/load"
            # "Child Instrument"
            # "typedef from Child Instrument"
            # "do not delete - used by framework"
            # "Data names and types of shift register data are defined by this bundle."
            # "Initialize the shift-register data, here.\n(data names are defined by what you wire into the bundle function)"
            n65 = call <userlib>:"Read Instrument.vi"("error in (no error)"=w181, "Instrument UI in"=w184) -> ("error out"=w182:errorcluster, "Instrument"=w183:refnum<class "Instrument.lvclass">, "Instrument UI"=w185:refnum<class "Inst UI.Krohn-Hite-7008.lvclass">)  [unwired: 7 in]
            n66 = To More Specific Class(target class=w194, reference=w183, error in=w182) -> (specific class reference=w193:refnum<class "Inst.Krohn-Hite-7008.lvclass">, error out=w192:errorcluster)
            n67 = Bundle("Core"=w195, "Instrument UI"=w185, "Instrument"=w193, "Configuration"=w191, "Message"=w190, "allChannelProperties"=w189, "Device"=w186, "Edit State"=w188, "Timer Reset"=w187) -> (w197:T16)  [unwired: 1 in]
            n68 = call <vilib>:"Add State(s) to Queue__jki_lib_state_machine.vi"("State(s) in (\"\")"=w199) -> ("States Out"=w198:string)  [unwired: 14 in]
          }
          frame "Data: Set UI Cluster" {
            # "Do not put any code in this frame.\n(It is a separator no-op. You can make a copy of this frame to create a new Data frame)"
            n69 = call <vilib>:"Add State(s) to Queue__jki_lib_state_machine.vi"("State(s) in (\"\")"=w204) -> ("States Out"=w203:string)  [unwired: 14 in]
          }
          frame "Data: Edit State" {
            # "Data: Edit State\n(Set Edit State == TRUE or FALSE)"
            n70 = Scan From String(input string=w209, default 1=FALSE ("Edit?")) -> (output 1=w205:bool)  [unwired: 3 in, 3 out]
            n71 = Bundle By Name(cluster=w206, "Edit State"=w205) -> (w207:T16)
            n72 = property on="Update" class="Bool (strict)"("Visible"=w205) -> ()  [unwired: 2 in, 2 out]
            n73 = property on="Cancel" class="Bool (strict)"("Visible"=w205) -> ()  [unwired: 2 in, 2 out]
            n74 = property on="Slide" class="Slide (strict)"("Visible"=w205) -> ()  [unwired: 2 in, 2 out]
            n75 = call <vilib>:"Add State(s) to Queue__jki_lib_state_machine.vi"("State(s) in (\"\")"=w213) -> ("States Out"=w212:string)  [unwired: 14 in]
          }
          frame "Data: Timer Reset" {
            # "Data: Timer Reset\n(Set Timer Reset == TRUE or FALSE)"
            n76 = Scan From String(input string=w218, default 1=FALSE ("Edit?")) -> (output 1=w216:bool)  [unwired: 3 in, 3 out]
            n77 = Bundle By Name(cluster=w214, "Timer Reset"=w216) -> (w215:T16)
            n78 = call <vilib>:"Add State(s) to Queue__jki_lib_state_machine.vi"("State(s) in (\"\")"=w222) -> ("States Out"=w221:string)  [unwired: 14 in]
          }
          frame "Data: Parse getAll" {
            # "Parse getAll"
            n79 = Unbundle By Name(w224) -> ("allChannelProperties"=w223:T1, "Message.Command"=w226:string, "Message.Data"=w230:variant)
            n80 = case shown="\"getAll\"" w226 {
              tunnel: w230 -> [_ w241]
              tunnel: [w234 w237] -> w225
              tunnel: [w235 w240] -> w228
              tunnel: w227 -> [w235 w239]
              tunnel: w223 -> [w234 _]
              frame Default {
              }
              frame "getAll" {
                n81 = Variant To Data(error in=w239, type=T11 {"allChannelProperties"=[{"channel"=1, "gain"=enum."10", "input"=enum."OFF", "shunt"=enum."10M", "couple"=enum."AC", "filter"=enum."OFF"}, {"channel"=2, "gain"=enum."10", "input"=enum."OFF", "shunt"=enum."10M", "couple"=enum."AC", "filter"=enum."OFF"}, {"channel"=3, "gain"=enum."10", "input"=enum."OFF", "shunt"=enum."10M", "couple"=enum."AC", "filter"=enum."OFF"}, {"channel"=4, "gain"=enum."10", "input"=enum."OFF", "shunt"=enum."10M", "couple"=enum."AC", "filter"=enum."OFF"}, {"channel"=5, "gain"=enum."10", "input"=enum."OFF", "shunt"=enum."10M", "couple"=enum."AC", "filter"=enum."OFF"}, {"channel"=6, "gain"=enum."10", "input"=enum."OFF", "shunt"=enum."10M", "couple"=enum."AC", "filter"=enum."OFF"}, {"channel"=7, "gain"=enum."10", "input"=enum."OFF", "shunt"=enum."10M", "couple"=enum."AC", "filter"=enum."OFF"}, {"channel"=7, "gain"=enum."10", "input"=enum."OFF", "shunt"=enum."10M", "couple"=enum."AC", "filter"=enum."OFF"}]} ("getAllChannelsResponse"), Variant=w241) -> (data=w236:T11, error out=w240:errorcluster)
                n82 = Unbundle By Name(w236) -> ("allChannelProperties"=w237:T1)
              }
            }
            n83 = Bundle By Name(cluster=w224, "allChannelProperties"=w225) -> (w229:T16)
            n84 = call <vilib>:"Add State(s) to Queue__jki_lib_state_machine.vi"("State(s) in (\"\")"=w233) -> ("States Out"=w232:string)  [unwired: 14 in]
          }
          frame "Data: Cleanup" {
            # "Cleanup any data and references, here.\n(this is called automatically, by the Macro: Exit)"
            n85 = Unbundle By Name(w242) -> ("Core.Current VI Reference"=w246:refnum<vi>)
            n86 = Close Reference(reference=w246, error in (no error)=w245) -> (error out=w244:errorcluster)
            n87 = call <vilib>:"Add State(s) to Queue__jki_lib_state_machine.vi"("State(s) in (\"\")"=w248) -> ("States Out"=w247:string)  [unwired: 14 in]
          }
          frame "---------- UI ----------" {
            # "Do not put any code in this frame.\n(It is a separator no-op. You can make a copy of this frame to create a new UI frame)"
            n88 = call <vilib>:"Add State(s) to Queue__jki_lib_state_machine.vi"("State(s) in (\"\")"=w253) -> ("States Out"=w252:string)  [unwired: 14 in]
          }
          frame "UI: Initialize" {
            w254 = FALSE ("Visible")
            # "size window to decoration box on front panel"
            # "Initialize the User Interface, here.\n(this is called automatically, by the Macro: Init)"
            n89 = invoke on="Cancel" class="Bool (strict)" method="Reinit To Default"() -> ()  [unwired: 3 in, 3 out]
            n90 = invoke on="Update" class="Bool (strict)" method="Reinit To Default"() -> ()  [unwired: 3 in, 3 out]
            n91 = invoke on="STOP" class="Bool (strict)" method="Reinit To Default"() -> ()  [unwired: 3 in, 3 out]
            n92 = call <userlib>:"Fit VI window to Largest Dec__ogtk.vi"("error in (no error)"=w257, "border spacing (2 px)"=0) -> ("error out"=w256:errorcluster)  [unwired: 4 in, 1 out]
            n93 = property on="Update" class="Bool (strict)"("Visible"=w254) -> ()  [unwired: 2 in, 2 out]
            n94 = property on="Cancel" class="Bool (strict)"("Visible"=w254) -> ()  [unwired: 2 in, 2 out]
            n95 = property on="Slide" class="Slide (strict)"("Visible"=w254) -> ()  [unwired: 2 in, 2 out]
            n96 = call <vilib>:"Add State(s) to Queue__jki_lib_state_machine.vi"("State(s) in (\"\")"=w261) -> ("States Out"=w260:string)  [unwired: 14 in]
          }
          frame "UI: Update FP Indicators" {
            n97 = Unbundle By Name(w273) -> ("Device.model"=w267:string, "Device.device_id"=w266:string, "allChannelProperties"=w272:T1, "Edit State"=w271:bool, "Instrument"=w263:refnum<class "Inst.Krohn-Hite-7008.lvclass">)
            n98 = call "Inst.KH7008.Read Index.vi"("error in (no error)"=w264, "Inst.Krohn-Hite-7008 in"=w263) -> ("error out"=w265:errorcluster, "Index"=w262:i32)  [unwired: 7 in, 1 out]
            n99 = call <userlib>:"MGI Get Executable Version.vi"() -> ("Version"=w268:string)  [unwired: 7 in]
            n100 = Format Into String(format string="%s #%d s/n %s\nApplication v%s", w267, w262, w266, w268) -> (resulting string=→"device":string)  [unwired: 2 in, 1 out]
            n101 = case shown="False" w271 {
              tunnel: w272 -> [w277 _]
              frame False {
                n102 = local write "allChannelProperties"(w277) -> ()
              }
              frame True {
              }
            }
            n103 = call <vilib>:"Add State(s) to Queue__jki_lib_state_machine.vi"("State(s) in (\"\")"=w276) -> ("States Out"=w275:string)  [unwired: 14 in]
          }
          frame "UI: Timer" {
            w292 = u32 60000 ("time (ms)")
            # "UI: Timer\n()"
            n104 = Unbundle By Name(w289) -> ("Edit State"=w278:bool, "Timer Reset"=w287:bool)
            n105 = call <userlib>:"Periodic Trigger__ogtk.vi"("time (ms)"=w292, "reset"=w287) -> ("Triggered"=w281:bool, "timer value"=w297:u32)  [unwired: 11 in, 1 out]
            n106 = To Long Integer(number=w292) -> (32bit integer=w295:i32)
            n107 = To Long Integer(number=w297) -> (32bit integer=w294:i32)
            n108 = Subtract(x=w295, y=w294) -> (x-y=w296:i32)
            n109 = Select(t=w296, s=w278, f=-60000) -> (s? t:f=w285:i32)
            "Slide" <- w285
            n110 = Quotient & Remainder(x=w285, y=1000) -> (floor(x/y)=w283:i32)  [unwired: 1 out]
            n111 = Format Into String(format string="Editing channelProperties. Push \"Update\" to commit, or reverting in %d s..." ("String"), w283) -> (resulting string=w280:string)  [unwired: 2 in, 1 out]
            n112 = Select(t=w280, s=w278, f="") -> (s? t:f=→"String":string)
            n113 = Select(t="Data: Edit State >> FALSE" ("State(s) in Front (\"\")"), s=w281, f="Data: Timer Reset >> FALSE" ("State(s) in Front (\"\")")) -> (s? t:f=w288:string)
            n114 = call <vilib>:"Add State(s) to Queue__jki_lib_state_machine.vi"("State(s) in Front (\"\")"=w288, "State(s) in (\"\")"=w301) -> ("States Out"=w300:string)  [unwired: 13 in]
          }
          frame "UI: SR Disable" {
            # "Do not put any code in this frame.\n(It is a separator no-op. You can make a copy of this frame to create a new UI frame)"
            n115 = control-ref of="channelProperties"() -> (w310:refnum<vi>)
            n116 = property class="Clust (strict)"(reference=w310) -> ("Controls[]"=w304:refnum<vi>[])  [unwired: 1 in, 2 out]
            n117 = for {
              tunnel: w304 -> [w318] mode=indexing
              tunnel: [w315] -> w305
              stop <- w314 stop-if-true
              n118 = property class="Ctl"(reference=w318) -> (reference out=w315:refnum<vi>, "Label.Text"=w317:string)  [unwired: 1 in, 1 out]
              n119 = Equal?(x=w317, y="shunt") -> (x = y?=w314:bool)
            }
            n120 = To More Specific Class(target class=refnum<vi> refnum ("specific class reference"), reference=w305) -> (specific class reference=w302:refnum<vi>)  [unwired: 1 in, 1 out]
            n121 = call "SR Disable.vi"("error in"=w308, "SR"=w306, "specific class reference"=w302) -> ("error out"=w309:errorcluster)  [unwired: 8 in]
            n122 = call <vilib>:"Add State(s) to Queue__jki_lib_state_machine.vi"("State(s) in (\"\")"=w313) -> ("States Out"=w312:string)  [unwired: 14 in]
          }
          frame "UI: Cursor Set" {
            # "Argument"
            # "Initialize the User Interface, here.\n(this is called automatically, by the Macro: Init)"
            n123 = disable-structure shown="Default" {
              disable-tunnel: w321 -> [w326 w329]
              disable-tunnel: [w326 w328] -> w320
              disable-tunnel: w319 -> [_ w327]
              frame condition #0 {
              }
              frame condition #1 (active) {
                n124 = case shown="\"Busy\"" w327 {
                  tunnel: w329 -> [w331 w333]
                  tunnel: [w330 w332] -> w328
                  frame "Idle", Default {
                    n125 = call <vilib>:"Unset Busy.vi"("error in (no error)"=w331) -> ("error out"=w330:errorcluster)  [unwired: 10 in]
                  }
                  frame "Busy" {
                    n126 = call <vilib>:"Set Busy.vi"("error in (no error)"=w333) -> ("error out"=w332:errorcluster)  [unwired: 9 in, 1 out]
                  }
                }
              }
            }
            n127 = call <vilib>:"Add State(s) to Queue__jki_lib_state_machine.vi"("State(s) in (\"\")"=w325) -> ("States Out"=w324:string)  [unwired: 14 in]
          }
          frame "UI: Front Panel State" {
            # "Argument"
            # "Set Front Panel Open or Closed\n(Usage: \"UI: Front Panel State >> Open|Close\")"
            n128 = Unbundle By Name(w337) -> ("Core.Current VI Reference"=w336:refnum<vi>)
            n129 = disable-structure shown="Default" {
              disable-tunnel: w339 -> [w345 w368]
              disable-tunnel: [w344 w368] -> w338
              disable-tunnel: w336 -> [w343 _]
              disable-tunnel: w335 -> [w342 _]
              frame condition #0 (active) {
                n130 = case shown="\"Close\"" w342 {
                  tunnel: w345 -> [w349 w362]
                  tunnel: [w351 w363] -> w344
                  tunnel: w343 -> [w350 w360]
                  frame "Open", Default {
                    n131 = property class="VI"(reference=w350, error in=w349) -> (reference out=w347:refnum<vi>, error out=w348:errorcluster, "FP.State"=w346:T12)
                    n132 = case shown="\"Closed\"" w346 {
                      tunnel: [w354 w357] -> w351
                      tunnel: w348 -> [w353 w357]
                      tunnel: w347 -> [w352 _]
                      frame "Closed" {
                        n133 = invoke class="VI" method="FP.Open"(reference=w352, error in=w353, "Activate"=TRUE, "State"=T12."Standard") -> (error out=w354:errorcluster)  [unwired: 1 in, 4 out]
                      }
                      frame Default {
                      }
                    }
                  }
                  frame "Close" {
                    n134 = property class="VI"(reference=w360, error in=w362) -> (reference out=w359:refnum<vi>, error out=w361:errorcluster, "FP.State"=w358:T12)
                    n135 = case shown="Default" w358 {
                      tunnel: [w364 w367] -> w363
                      tunnel: w361 -> [w364 w366]
                      tunnel: w359 -> [_ w365]
                      frame "Invalid", "Closed" {
                      }
                      frame Default {
                        n136 = invoke class="VI" method="FP.Close"(reference=w365, error in=w366) -> (error out=w367:errorcluster)  [unwired: 1 in, 2 out]
                      }
                    }
                  }
                }
              }
              frame condition #1 {
              }
            }
            n137 = call <vilib>:"Add State(s) to Queue__jki_lib_state_machine.vi"("State(s) in (\"\")"=w341) -> ("States Out"=w340:string)  [unwired: 14 in]
          }
          frame "---------- Macro ----------" {
            # "Do not put any code in this frame.\n(It is a separator no-op. You can make a copy of this frame to create a new Macro frame)"
            n138 = call <vilib>:"Add State(s) to Queue__jki_lib_state_machine.vi"("State(s) in (\"\")"=w373) -> ("States Out"=w372:string)  [unwired: 14 in]
          }
          frame "Macro: Initialize" {
            # "Initialization Macro\n(This is called once, when the VI starts)"
            n139 = call <vilib>:"Add State(s) to Queue__jki_lib_state_machine.vi"("State(s) in Front (\"\")"="Data: Initialize\nInitialize Core Data\nEvents: Register", "State(s) in (\"\")"="Process: Sync", "State(s) at Back (\"\")"="UI: Initialize\nMacro: Read UI Config\nAction: Wait >> 2000\nAction: Open\nAction: IDN") -> ("States Out"=w375:string)  [unwired: 12 in]
            n140 = call <vilib>:"Add State(s) to Queue__jki_lib_state_machine.vi"("State(s) in Front (\"\")"=w375, "State(s) in (\"\")"=w382) -> ("States Out"=w381:string)  [unwired: 13 in]
          }
          frame "Macro: Post Error Handling" {
            # "Clear Last Error?"
            n141 = Unbundle By Name(w384) -> ("Core.Last Error.remaining states"=w386:string, "Core.Shutdown?"=w387:bool)
            n142 = Unbundle By Name(w384) -> ("Core.Last Error.error"=w390:errorcluster)
            n143 = case shown="False" FALSE {
              tunnel: w390 -> [w398 _]
              tunnel: [w398 _] -> w389
              frame False {
              }
              frame True {
              }
            }
            n144 = case shown="True" w387 {
              tunnel: w386 -> [w395 w397]
              tunnel: [w395 w396] -> w383
              frame False {
                # "These are the remaining states (at the moment the error occured). States can be altered according to business logic."
                # "NOT SHUTTING DOWN"
              }
              frame True {
                # "Developer can decide to alter the states but should be aware that during the shutdown process, there are certain states that must be run for the SMO to properly shut itself (and this process) down. As such, one can add states to perform additional clean-ups, but should append the remaining state to be executed."
                # "SHUTTING DOWN"
                n145 = call <vilib>:"Add State(s) to Queue__jki_lib_state_machine.vi"("State(s) in (\"\")"=w397) -> ("States Out"=w396:string)  [unwired: 14 in]
              }
            }
            n146 = Bundle By Name(cluster=w384, "Core.Last Error.error"=w389) -> (w385:T16)
            n147 = call <vilib>:"Add State(s) to Queue__jki_lib_state_machine.vi"("State(s) in Front (\"\")"=w383, "State(s) in (\"\")"=w394) -> ("States Out"=w393:string)  [unwired: 13 in]
          }
          frame "Macro: Read UI Config" {
            # "Do not put any code in this frame.\n(It is a separator no-op. You can make a copy of this frame to create a new Macro frame)"
            n148 = call <vilib>:"Add State(s) to Queue__jki_lib_state_machine.vi"("State(s) in Front (\"\")"="Configuration: Initialize\nConfiguration: Read UI Config File" ("State(s) in Front (\"\")"), "State(s) in (\"\")"=w404) -> ("States Out"=w403:string)  [unwired: 13 in]
          }
          frame "Macro: Write UI Config" {
            # "Do not put any code in this frame.\n(It is a separator no-op. You can make a copy of this frame to create a new Macro frame)"
            n149 = call <vilib>:"Add State(s) to Queue__jki_lib_state_machine.vi"("State(s) in Front (\"\")"="Data: Set UI Cluster\nConfiguration: Write UI Config File" ("State(s) in Front (\"\")"), "State(s) in (\"\")"=w410) -> ("States Out"=w409:string)  [unwired: 13 in]
          }
          frame "Macro: Exit" {
            # "Exit Macro\n(This is called once, when the VI exits)"
            n150 = Unbundle By Name(w412) -> ("Core.Close Panel on Exit?"=w422:bool)
            n151 = Select(t="UI: Front Panel State >> Close", s=w422, f="" ("Empty String Constant")) -> (s? t:f=w419:string)
            n152 = call <vilib>:"Add State(s) to Queue__jki_lib_state_machine.vi"("State(s) in Front (\"\")"="Data: Cleanup\nEvents: Unregister\nProcess: Self Terminate", "State(s) in (\"\")"="Process: Sync", "State(s) at Back (\"\")"="Exit") -> ("States Out"=w414:string)  [unwired: 12 in]
            n153 = call <vilib>:"Add State(s) to Queue__jki_lib_state_machine.vi"("State(s) in Front (\"\")"="//Action: Close\nMacro: Write UI Config", "State(s) in (\"\")"=w419, "State(s) at Back (\"\")"=w414) -> ("States Out"=w418:string)  [unwired: 12 in]
            n154 = call <vilib>:"Add State(s) to Queue__jki_lib_state_machine.vi"("State(s) in Front (\"\")"=w418, "State(s) in (\"\")"=w425) -> ("States Out"=w424:string)  [unwired: 13 in]
          }
          frame "---------- Process ----------" {
            # "Template Separator\n(You can make a copy of, or modify, this frame)"
            n155 = call <vilib>:"Add State(s) to Queue__jki_lib_state_machine.vi"("State(s) in (\"\")"=w430) -> ("States Out"=w429:string)  [unwired: 14 in]
          }
          frame "Process: Sync" {
            n156 = Unbundle By Name(w438) -> ("Instrument UI"=w434:refnum<class "Inst UI.Krohn-Hite-7008.lvclass">)
            n157 = call <vilib>:"WaitOnProcessSync.vi"("error in (no error)"=w433, "SMO"=w434) -> ("error out"=w432:errorcluster, "Don't run?"=w437:bool)  [unwired: 7 in, 1 out]
            n158 = Select(t="Data: Cleanup\nEvents: Unregister\nExit", s=w437, f="" ("Empty String Constant")) -> (s? t:f=w431:string)
            n159 = call <vilib>:"Add State(s) to Queue__jki_lib_state_machine.vi"("State(s) in Front (\"\")"=w431, "State(s) in (\"\")"=w441) -> ("States Out"=w440:string)  [unwired: 13 in]
          }
          frame "Process: Self Terminate" {
            n160 = Unbundle By Name(w443) -> ("Instrument UI"=w442:refnum<class "Inst UI.Krohn-Hite-7008.lvclass">)
            n161 = call <vilib>:"SelfTerminate.vi"("error in (no error)"=w445, "SMO in"=w442) -> ("error out"=w444:errorcluster)  [unwired: 8 in, 1 out]
            n162 = call <vilib>:"Add State(s) to Queue__jki_lib_state_machine.vi"("State(s) in (\"\")"=w448) -> ("States Out"=w447:string)  [unwired: 14 in]
          }
          frame "---------- Events ----------" {
            # "Template Separator\n(You can make a copy of, or modify, this frame)"
            n163 = call <vilib>:"Add State(s) to Queue__jki_lib_state_machine.vi"("State(s) in (\"\")"=w453) -> ("States Out"=w452:string)  [unwired: 14 in]
          }
          frame "Events: Register" {
            # "Expand to add\nmore events"
            # "Base Class Protected Events"
            n164 = Unbundle By Name(w467) -> ("Instrument UI"=w460:refnum<class "Inst UI.Krohn-Hite-7008.lvclass">, "Instrument"=w459:refnum<class "Inst.Krohn-Hite-7008.lvclass">)
            n165 = call <vilib>:"GetProtectedEvents.vi"("SMO"=w460) -> ("error out"=w463:errorcluster, "SMO Protected Events"=w465:T21)  [unwired: 8 in, 1 out]
            n166 = call <userlib>:"Instrument.GetPublicEvents.vi"("Instrument"=w459) -> ("error out"=w461:errorcluster, "Instrument Public Events"=w462:T22, "Instrument out"=w457:refnum<class "Inst.Krohn-Hite-7008.lvclass">)  [unwired: 8 in]
            n167 = call "Inst.KH7008.GetPublicEvents.vi"("Inst.Krohn-Hite-7008 in"=w457) -> ("error out"=w456:errorcluster, "Inst.Krohn-Hite-7008 Public Events"=w458:T23)  [unwired: 8 in, 1 out]
            n168 = register-events(w465, w462, w458) -> (reference out=w466:refnum<event-registration>, error out=w455:errorcluster)  [unwired: 2 in]
            n169 = Merge Errors(w455, w456, w461, w463, w454) -> (w464:errorcluster)
            n170 = call <vilib>:"Add State(s) to Queue__jki_lib_state_machine.vi"("State(s) in (\"\")"=w469) -> ("States Out"=w468:string)  [unwired: 14 in]
          }
          frame "Events: Unregister" {
            n171 = Unregister For Events(event registration refnum=w472, error in=w471) -> (error out=w470:errorcluster)
            n172 = call <vilib>:"Add State(s) to Queue__jki_lib_state_machine.vi"("State(s) in (\"\")"=w475) -> ("States Out"=w474:string)  [unwired: 14 in]
          }
          frame "---------- Configuration ----------" {
            # "Do not put any code in this frame.\n(It is a separator no-op. You can make a copy of this frame to create a new UI frame)"
            n173 = call <vilib>:"Add State(s) to Queue__jki_lib_state_machine.vi"("State(s) in (\"\")"=w480) -> ("States Out"=w479:string)  [unwired: 14 in]
          }
          frame "Configuration: Initialize" {
            # "Do not put any code in this frame.\n(It is a separator no-op. You can make a copy of this frame to create a new UI frame)"
            n174 = Unbundle By Name(w488) -> ("Configuration"=w486:refnum<class "Configuration.lvclass">, "Instrument"=w487:refnum<class "Inst.Krohn-Hite-7008.lvclass">)
            n175 = call <vilib>:"GetName.vi"("error in (no error)"=w490, "SMO"=w487) -> ("error out"=w489:errorcluster, "Name"=w491:string)  [unwired: 6 in, 2 out]
            n176 = call <userlib>:"Default Path.vi"("error in (no error)"=w489, "Folder Name [Application Name]"=w491, "Configuration in"=w486) -> ("error out"=w482:errorcluster, "Configuration out"=w485:refnum<class "Configuration.lvclass">)  [unwired: 7 in]
            n177 = call <userlib>:"Write Section.vi"("error in (no error)"=w482, "Section"="UI", "Configuration in"=w485) -> ("error out"=w481:errorcluster, "Configuration out"=w484:refnum<class "Configuration.lvclass">)  [unwired: 7 in]
            n178 = Bundle By Name(cluster=w488, "Configuration"=w484) -> (w492:T16)
            n179 = call <vilib>:"Add State(s) to Queue__jki_lib_state_machine.vi"("State(s) in (\"\")"=w495) -> ("States Out"=w494:string)  [unwired: 14 in]
          }
          frame "Configuration: Write UI Config File" {
            # "Do not put any code in this frame.\n(It is a separator no-op. You can make a copy of this frame to create a new Data frame)"
            n180 = Unbundle By Name(w500) -> ("Configuration"=w497:refnum<class "Configuration.lvclass">, "Message"=w499:T14)
            n181 = call <userlib>:"Write Configuration.vi"("error in (no error)"=w496, "Variant"=w499, "Configuration in"=w497) -> ("error out"=w498:errorcluster)  [unwired: 7 in, 1 out]
            n182 = call <vilib>:"Add State(s) to Queue__jki_lib_state_machine.vi"("State(s) in (\"\")"=w503) -> ("States Out"=w502:string)  [unwired: 14 in]
          }
          frame "Configuration: Read UI Config File" {
            # "Do not put any code in this frame.\n(It is a separator no-op. You can make a copy of this frame to create a new UI frame)"
            n183 = Unbundle By Name(w506) -> ("Message"=w509:T14, "Configuration"=w512:refnum<class "Configuration.lvclass">)
            n184 = call <userlib>:"Read Configuration.vi"("INI Fomatted Cluster Type"=w509, "error in (no error)"=w508, "Configuration in"=w512) -> ("error out"=w511:errorcluster, "Configuration"=w510:variant)  [unwired: 6 in, 1 out]
            n185 = Variant To Data(error in=w511, type=w509, Variant=w510) -> (data=w505:T14, error out=w507:errorcluster)
            n186 = Bundle By Name(cluster=w506, "Message"=w505) -> (w504:T16)
            n187 = call <vilib>:"Add State(s) to Queue__jki_lib_state_machine.vi"("State(s) in (\"\")"=w515) -> ("States Out"=w514:string)  [unwired: 14 in]
          }
          frame "---------- Action ----------" {
            n188 = Unbundle By Name(w517) -> ("Instrument"=w518:refnum<class "Inst.Krohn-Hite-7008.lvclass">)
            n189 = Bundle By Name(cluster=w517, "Instrument"=w518) -> (w516:T16)
            n190 = call <vilib>:"Add State(s) to Queue__jki_lib_state_machine.vi"("State(s) in (\"\")"=w522) -> ("States Out"=w521:string)  [unwired: 14 in]
          }
          frame "Action: Notify UI Closed" {
            # "Notify that the UI has been closed"
            n191 = Unbundle By Name(w523) -> ("Instrument UI"=w526:refnum<class "Inst UI.Krohn-Hite-7008.lvclass">)
            n192 = call <vilib>:"Hide.vi"("error in (no error)"=w525, "SMO.UI"=w526) -> ("error out"=w524:errorcluster)  [unwired: 8 in, 1 out]
            n193 = call <vilib>:"Add State(s) to Queue__jki_lib_state_machine.vi"("State(s) in (\"\")"=w529) -> ("States Out"=w528:string)  [unwired: 14 in]
          }
          frame "Action: Open" {
            n194 = Unbundle By Name(w536) -> ("Instrument"=w534:refnum<class "Inst.Krohn-Hite-7008.lvclass">)
            n195 = call <userlib>:"Write Client Type.vi"("error in (no error)"=w531, "Client Type [Remote]"=Client_Type--Enum."Local" ("Client Type"), "Instrument in"=w534) -> ("error out"=w532:errorcluster, "Instrument out"=w533:refnum<class "Inst.Krohn-Hite-7008.lvclass">)  [unwired: 7 in]
            n196 = call-dynamic "Open.vi"("error in (no error)"=w532, "Inst.Krohn-Hite-7008 in"=w533) -> ("error out"=w539:errorcluster, "Inst.Krohn-Hite-7008 out"=w535:refnum<class "Inst.Krohn-Hite-7008.lvclass">)  [unwired: 8 in]
            n197 = Bundle By Name(cluster=w536, "Instrument"=w535) -> (w537:T16)
            n198 = call <vilib>:"Add State(s) to Queue__jki_lib_state_machine.vi"("State(s) in Front (\"\")"="" ("State(s) in Front (\"\")"), "State(s) in (\"\")"=w542) -> ("States Out"=w541:string)  [unwired: 13 in]
          }
          frame "Action: IDN" {
            n199 = Unbundle By Name(w552) -> ("Instrument"=w550:refnum<class "Inst.Krohn-Hite-7008.lvclass">)
            n200 = call <userlib>:"IDN.vi"("error in (no error)"=w547, "Instrument in"=w550) -> ("error out"=w548:errorcluster, "IDN"=w546:T24, "Instrument in"=w549:refnum<class "Inst.Krohn-Hite-7008.lvclass">)  [unwired: 7 in]
            n201 = Unbundle By Name(w546) -> ("model"=w544:string, "serial"=w545:string)
            n202 = Bundle By Name(cluster=w552, "Instrument"=w549, "Device.model"=w544, "Device.device_id"=w545) -> (w551:T16)
            n203 = call <vilib>:"Add State(s) to Queue__jki_lib_state_machine.vi"("State(s) in Front (\"\")"="UI: Update FP Indicators" ("State(s) in Front (\"\")"), "State(s) in (\"\")"=w555) -> ("States Out"=w554:string)  [unwired: 13 in]
          }
          frame "Action: Close" {
            n204 = Unbundle By Name(w557) -> ("Instrument"=w560:refnum<class "Inst.Krohn-Hite-7008.lvclass">)
            n205 = call-dynamic "Close.vi"("error in (no error)"=w558, "Inst.Krohn-Hite-7008 in"=w560) -> ("error out"=w562:errorcluster, "Inst.Krohn-Hite-7008 out"=w556:refnum<class "Inst.Krohn-Hite-7008.lvclass">)  [unwired: 8 in]
            n206 = Bundle By Name(cluster=w557, "Instrument"=w556) -> (w559:T16)
            n207 = call <vilib>:"Add State(s) to Queue__jki_lib_state_machine.vi"("State(s) in Front (\"\")"="" ("State(s) in Front (\"\")"), "State(s) in (\"\")"=w565) -> ("States Out"=w564:string)  [unwired: 13 in]
          }
          frame "Action: Wait" {
            n208 = Unbundle By Name(w571) -> ("Instrument"=w572:refnum<class "Inst.Krohn-Hite-7008.lvclass">)
            n209 = Scan From String(format string="%d", input string=w566, default 1=u32 0 ("default value 1")) -> (output 1=w567:u32)  [unwired: 2 in, 3 out]
            n210 = Wait (ms)(milliseconds to wait=w567) -> ()  [unwired: 1 out]
            n211 = Bundle By Name(cluster=w571, "Instrument"=w572) -> (w570:T16)
            n212 = call <vilib>:"Add State(s) to Queue__jki_lib_state_machine.vi"("State(s) in (\"\")"=w576) -> ("States Out"=w575:string)  [unwired: 14 in]
          }
          frame "Action: setAllChannels" {
            # "Send a message (command, data, etc) to the Instrument:process.vi"
            n213 = Unbundle By Name(w582) -> ("Instrument"=w581:refnum<class "Inst.Krohn-Hite-7008.lvclass">, "allChannelProperties"=w577:T1)
            n214 = call-dynamic "Inst.KH7008.setAllChannels.vi"("error in (no error)"=w580, "allChannelProperties"=w577, "Inst.Krohn-Hite-7008 in"=w581) -> ("error out"=w579:errorcluster, "Inst.Krohn-Hite-7008 out"=w578:refnum<class "Inst.Krohn-Hite-7008.lvclass">)  [unwired: 7 in]
            n215 = Bundle By Name(cluster=w582, "Instrument"=w578) -> (w583:T16)
            n216 = call <vilib>:"Add State(s) to Queue__jki_lib_state_machine.vi"("State(s) in Front (\"\")"="" ("State(s) in Front (\"\")"), "State(s) in (\"\")"=w587) -> ("States Out"=w586:string)  [unwired: 13 in]
          }
          frame "Action: Send Message to Instrument" {
            # "\"local\""
            # "Send a message (command, data, etc) to the Instrument:process.vi"
            n217 = Unbundle By Name(w592) -> ("Instrument"=w591:refnum<class "Inst.Krohn-Hite-7008.lvclass">)
            n218 = call-poly <userlib>:"Instrument.sendMessageToProcess.vi"("error in (no error)"=w589, "Instrument"=w591) -> ("error out"=w588:errorcluster, "Instrument out"=w590:refnum<class "Inst.Krohn-Hite-7008.lvclass">)  [unwired: 8 in]
            n219 = Bundle By Name(cluster=w592, "Instrument"=w590) -> (w593:T16)
            n220 = call <vilib>:"Add State(s) to Queue__jki_lib_state_machine.vi"("State(s) in Front (\"\")"="" ("State(s) in Front (\"\")"), "State(s) in (\"\")"=w597) -> ("States Out"=w596:string)  [unwired: 13 in]
          }
          frame "Action: Send Message to Child" {
            # "Send a message (command, data, etc) to the Instrument.Child:process.vi"
            n221 = Unbundle By Name(w602) -> ("Instrument"=w601:refnum<class "Inst.Krohn-Hite-7008.lvclass">)
            n222 = call "Inst.KH7008.MessageToProcess.vi"("error in (no error)"=w599, "Inst.Krohn-Hite-7008 in"=w601) -> ("error out"=w598:errorcluster, "Inst.Krohn-Hite-7008 out"=w600:refnum<class "Inst.Krohn-Hite-7008.lvclass">)  [unwired: 8 in]
            n223 = Bundle By Name(cluster=w602, "Instrument"=w600) -> (w603:T16)
            n224 = call <vilib>:"Add State(s) to Queue__jki_lib_state_machine.vi"("State(s) in Front (\"\")"="" ("State(s) in Front (\"\")"), "State(s) in (\"\")"=w607) -> ("States Out"=w606:string)  [unwired: 13 in]
          }
        }
      }
    }
    frame Error {
    }
  }
  n225 = call-parent "Process.vi"("error in"=w5, "Instrument UI in"=w4) -> ("error out"=w2:errorcluster, "Instrument UI out"=→"Inst UI.Krohn-Hite-7008 out":refnum<class "Inst UI.Krohn-Hite-7008.lvclass">)  [unwired: 8 in]
  n226 = Merge Errors(w2, w1) -> (→"error out":errorcluster)
  n227 = disable-structure shown="Disabled" {
    frame Disabled {
      w609 = u32 500 ("time (ms)")
      # "#todo\nyou can put a timer on the front panel\nto show when it will refresh again"
      # "Call Action: getAll according to refresh time"
      n228 = call <userlib>:"Periodic Trigger__ogtk.vi"("time (ms)"=w609) -> ("Triggered"=w616:bool, "timer value"=w613:u32)  [unwired: 12 in, 1 out]
      n229 = Subtract(x=w609, y=w613) -> (x-y=w614:u32)
      n230 = In Range and Coerce(upper limit=w609, x=w614, lower limit=u32 0) -> (coerced(x)=→"Numeric":u32)  [unwired: 1 out]
      n231 = Select(t="//UI: Update FP Indicators" ("State(s) in Front (\"\")"), s=w616, f="UI: Timer" ("State(s) in Front (\"\")")) -> ()  [unwired: 1 out]
    }
    frame Enabled {
    }
  }
